vi "SimulatedTHD.vi"(8 "error in (no error)":errorcluster) -> (0 "error out":errorcluster, 2 "THD":cluster{"f0":dbl, "df":dbl, "magnitude":dbl[]} {"magnitude" format="%.2p"; "f0" format="%0.2p"; "df" format="%0.2p"})   [LabVIEW 2014]
doc: "This subVI is used to create a Sine, Square, Triangle or Sawtooth Waveform. The inputs to this VI are the Waveform Type, which determines if the output waveform is a Sine, Square, Triangle, or Sawtooth Waveform, the amplitude, Desired Frequency, Samples per Buffer, and Cycles per Buffer. \n\nThe Desired Frequency, Samples per Buffer, and Cycles per Buffer are used to calculate the sample clock rate. The DAQmx Timing property node sets the sample clock rate for the device specified in the task/channels in control. \n\nThe actual, coerced, sample clock rate is returned and used as an input to the Basic Function Generator.vi. The Basic Function Generator returns a waveform of data with timing information.\n\nThe formula below was used to determine the sample clock rate:\n\nDesired Frequency=[(Cycles/Buffer)X(Sample Clock Rate)]/Samples per Buffer\n\nNote: The Block Diagram rearranges the variables to solve for Sample Clock Rate"
uses:
  <vilib>/Analysis/4window.llb/windowTd.ctl
  <vilib>/measure/maspectr.llb/FFT Power Spectrum for 1 Chan.vi
  <vilib>/measure/NI_MABase.lvlib
  <vilib>/measure/NI_MAPro.lvlib
  <vilib>/Analysis/NI_AALPro.lvlib
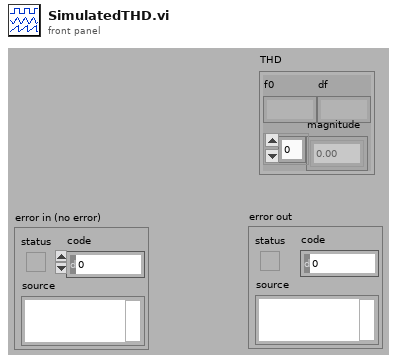
[diagram p1: front panel]
types:
  T1 = typedef "NI_AALPro.lvlib/windowTd.ctl" = u32
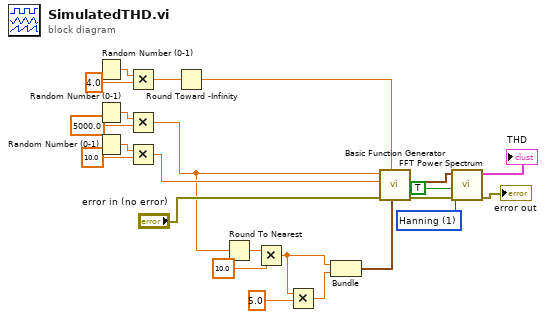
[diagram p0: block diagram]
diagram:
  w21 = T1 1 items=["Rectangle"=0, "Hanning"=1, "Hamming"=2, "Blackman-Harris"=3, "Exact Blackman"=4, "Blackman"=5, "Flat Top"=6, "4 Term B-Harris "=7, "7 Term B-Harris"=8, "Low Sidelobe"=9, "Blackman Nuttall"=11, "Triangle"=30, "Bartlett-Hanning"=31, "Bohman"=32, "Parzen"=33, "Welch"=34, "Kaiser"=60, "Dolph-Chebyshev"=61, "Gaussian"=62] ("window")
  n1 = Random Number (0-1)() -> (number: 0 to 1=w11:dbl)
  n2 = Random Number (0-1)() -> (number: 0 to 1=w12:dbl)
  n3 = Random Number (0-1)() -> (number: 0 to 1=w16:dbl)
  n4 = Multiply(x=w11, y=4.0) -> (x*y=w9:dbl)
  n5 = Multiply(x=w12, y=5000.0) -> (x*y=w7:dbl)
  n6 = Multiply(x=w16, y=10.0) -> (x*y=w14:dbl)
  n7 = Round Toward -Infinity(1:w9) -> (0:w8:dbl)
  n8 = Round To Nearest(number=w7) -> (nearest integer value=w6:dbl)
  n9 = Multiply(x=w6, y=10.0) -> (x*y=w2:dbl)
  n10 = Multiply(x=w2, y=5.0) -> (x*y=w3:dbl)
  n11 = Bundle(w2, w3) -> (w1:cluster{dbl, dbl})  [unwired: 1 in]
  n12 = call <vilib>:"Basic Function Generator.vi"("sampling info"=w1, "signal type"=w8, "error in (no error)"="error in (no error)", "amplitude"=w14, "frequency"=w7) -> ("error out"=w23:errorcluster, "signal out"=w19:waveform(dbl))  [unwired: 4 in, 1 out]
  n13 = call-poly <vilib>:"FFT Power Spectrum.vi"("error in (no error)"=w23, "dB On (F)"=TRUE, "window"=w21, "time signal"=w19) -> ("error out"=→"error out":errorcluster, "power spectrum"=→"THD":cluster{"f0":dbl, "df":dbl, "magnitude":dbl[]})  [unwired: 4 in, 2 out]
